vi "Network Error.vi"(8 "error in (no error)":errorcluster, 9 "String to Append":string, 10 "Error":T1, 11 "Insert Error":bool=TRUE) -> (0 "error out":errorcluster)   [LabVIEW 2021, in "Networking_CIF_U.lvlib"]
uses:
  Networking_CIF_U.lvlib
  Typedef/Errors.ctl
  Errors/Errors_CIF_U.lvlib
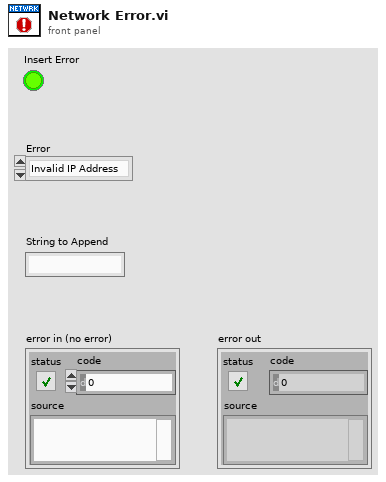
[diagram p1: front panel]
types:
  T1 = typedef "Networking_CIF_U.lvlib/Errors.ctl" = enum16{"Invalid IP Address", "No Subnet Match Found", "Error Finding Port", "No Ping Response", "Nettools Needed"}
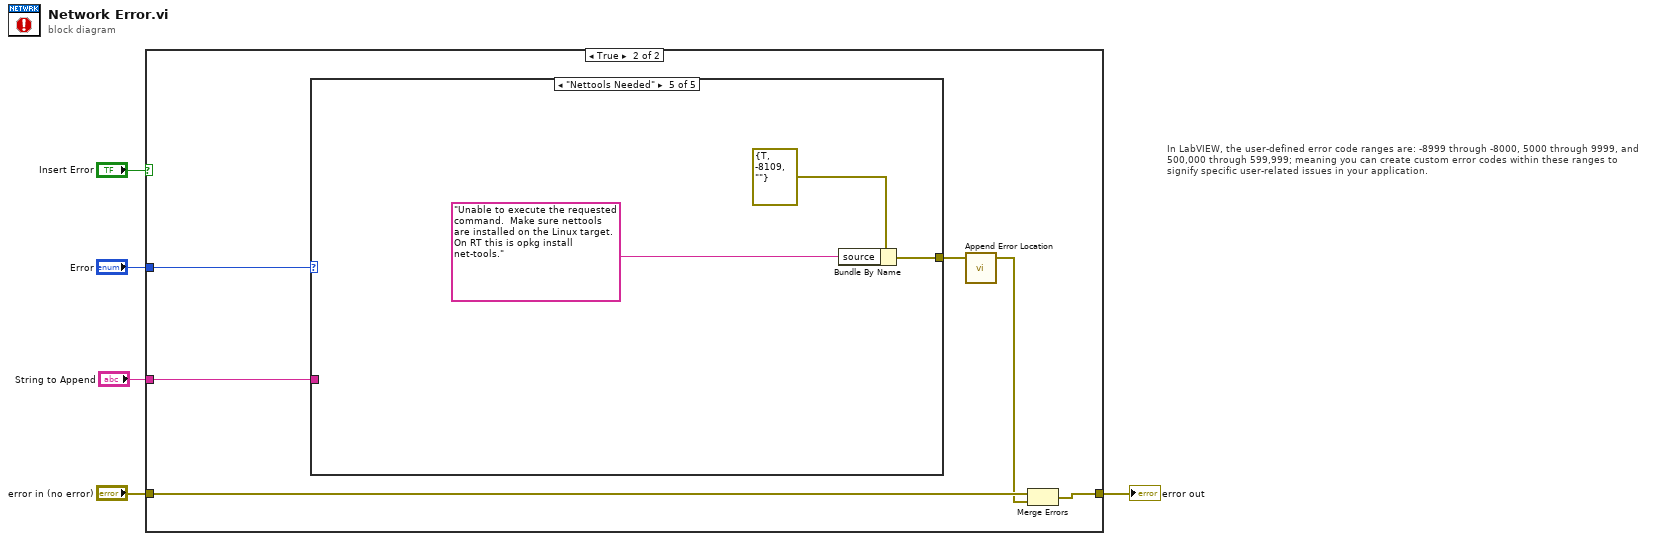
[diagram p0: block diagram]
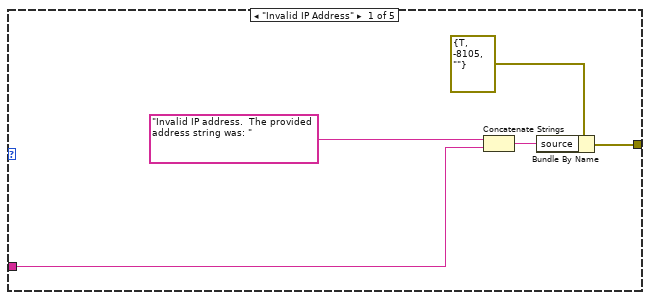
[diagram p3: hidden frame]
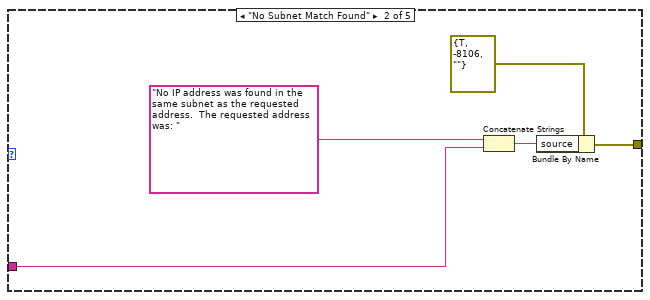
[diagram p4: hidden frame]
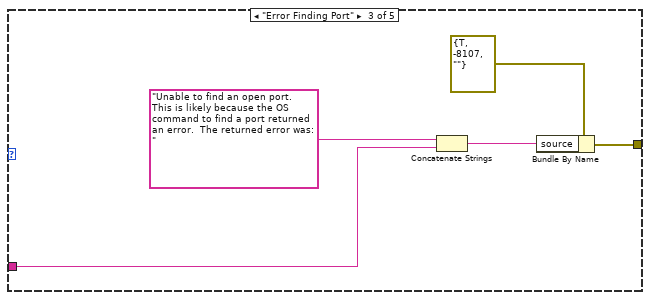
[diagram p5: hidden frame]
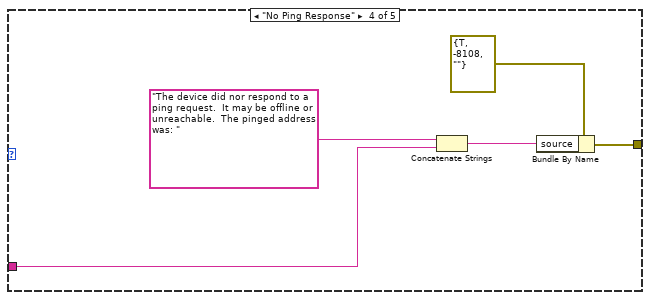
[diagram p6: hidden frame]
diagram:
  # "In LabVIEW, the user-defined error code ranges are: -8999 through -8000, 5000 through 9999, and 500,000 through 599,999; meaning you can create custom error codes within these ranges to signify specific user-related issues in your application."
  n1 = case shown="True" "Insert Error" {
    tunnel: [w6 w9] -> w4
    tunnel: "error in (no error)" -> [w6 w10]
    tunnel: "Error" -> [_ w12]
    tunnel: "String to Append" -> [_ w11]
    frame False {
    }
    frame True {
      n2 = case shown="\"Nettools Needed\"" w12 {
        tunnel: w11 -> [w14 w19 w23 w28 _]
        tunnel: [w16 w21 w26 w31 w34] -> w8
        frame "Invalid IP Address" {
          n3 = Concatenate Strings("Invalid IP address.  The provided address string was: " ("source"), w14) -> (w13:string)
          n4 = Bundle By Name(cluster=errorcluster {"status"=TRUE, "code"=-8105, "source"=""} ("Invalid ID"), "source"=w13) -> (w16:errorcluster)
        }
        frame "No Subnet Match Found" {
          n5 = Concatenate Strings("No IP address was found in the same subnet as the requested address.  The requested address was: " ("source"), w19) -> (w18:string)
          n6 = Bundle By Name(cluster=errorcluster {"status"=TRUE, "code"=-8106, "source"=""} ("Invalid ID"), "source"=w18) -> (w21:errorcluster)
        }
        frame "Error Finding Port" {
          n7 = Concatenate Strings("Unable to find an open port.  This is likely because the OS command to find a port returned an error.  The returned error was: " ("source"), w23) -> (w24:string)
          n8 = Bundle By Name(cluster=errorcluster {"status"=TRUE, "code"=-8107, "source"=""} ("Invalid ID"), "source"=w24) -> (w26:errorcluster)
        }
        frame "No Ping Response" {
          n9 = Concatenate Strings("The device did nor respond to a ping request.  It may be offline or unreachable.  The pinged address was: " ("source"), w28) -> (w29:string)
          n10 = Bundle By Name(cluster=errorcluster {"status"=TRUE, "code"=-8108, "source"=""} ("Invalid ID"), "source"=w29) -> (w31:errorcluster)
        }
        frame "Nettools Needed" {
          n11 = Bundle By Name(cluster=errorcluster {"status"=TRUE, "code"=-8109, "source"=""} ("Invalid ID"), "source"="Unable to execute the requested command.  Make sure nettools are installed on the Linux target.   On RT this is opkg install net-tools.") -> (w34:errorcluster)
        }
      }
      n12 = call "Append Error Location.vi"("error in (no error)"=w8) -> ("error out"=w7:errorcluster)  [unwired: 4 in]
      n13 = Merge Errors(w10, w7) -> (w9:errorcluster)
    }
  }
  "error out" <- w4
